vi "Get Startup Requirements.vi"(8 "error in (no error)":errorcluster, 10 "Startup Component":T1={"title"="", "description"="", "ID"="", "version"="", "component type"=4} {"component type" items=["standard", "hidden", "system", "unknown", "startup", "image", "essential"]}, 11 "Session in":refnum<k21>) -> (0 "error out":errorcluster, 1 "Software Set":T3 {"information"."component type" items=["standard", "hidden", "system", "unknown", "startup", "image", "essential"]; "items"."component type" items=["standard", "hidden", "system", "unknown", "startup", "image", "essential"]; "add-ons"."component type" items=["standard", "hidden", "system", "unknown", "startup", "image", "essential"]}, 2 "Dependencies":T4[](array[typedef]) {"dependee"."component type" items=["standard", "hidden", "system", "unknown", "startup", "image", "essential"]; "depender"."component type" items=["standard", "hidden", "system", "unknown", "startup", "image", "essential"]}, 3 "Session out":refnum<k21>)   [LabVIEW 2017, in "nisyscfg.lvlib"]
uses:
  <vilib>/nisyscfg/nisyscfg.lvlib
  <vilib>/nisyscfg/Broken Dependency 1.2.ctl
  <vilib>/nisyscfg/Software 1.2.ctl
  <vilib>/nisyscfg/Component Type.ctl
  <vilib>/nisyscfg/Software Set 1.2.ctl
  <vilib>/nisyscfg/Component Types.ctl
panel:
  out "Visibility Type":u32
  out "Type":u32
  out "Number of Items":i32
  out "Items":u64
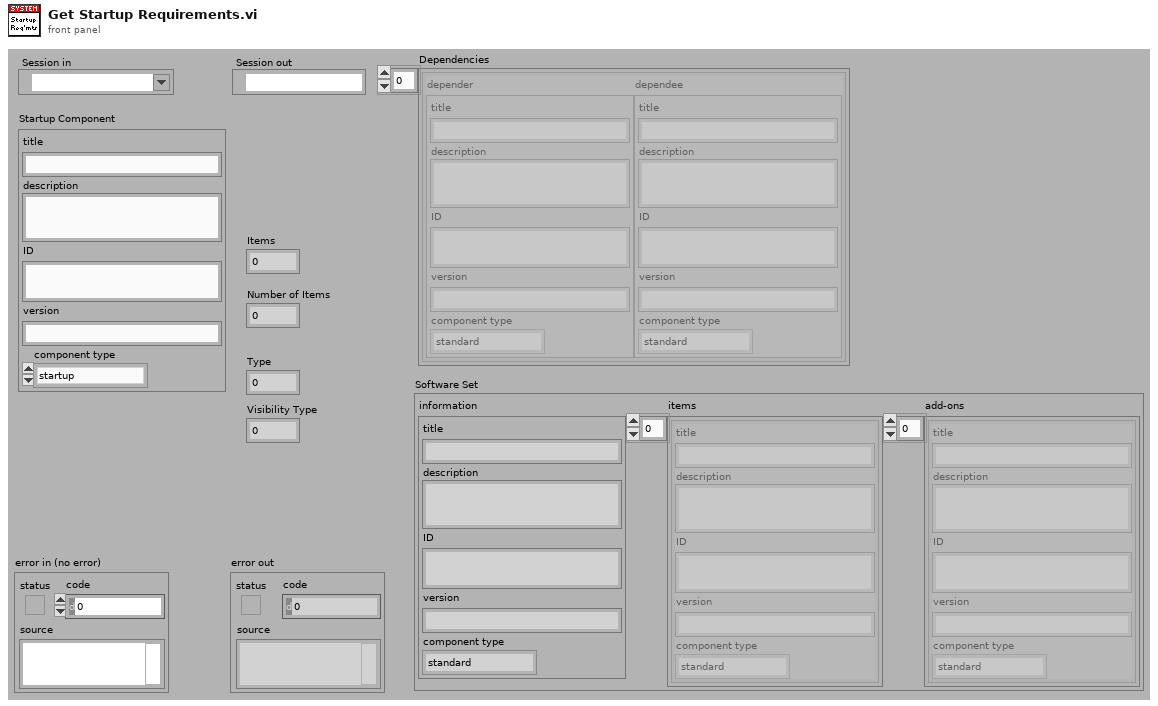
[diagram p1: front panel]
types:
  T1 = typedef "nisyscfg.lvlib/Software 1.2.ctl" = cluster{"title":string, "description":string, "ID":string, "version":string, "component type":T2}
  T2 = typedef "nisyscfg.lvlib/Component Type.ctl" = u32
  T3 = typedef "nisyscfg.lvlib/Software Set 1.2.ctl" = cluster{"information":T1, "items":T1[], "add-ons":T1[]}
  T4 = typedef "nisyscfg.lvlib/Broken Dependency 1.2.ctl" = cluster{"depender":T1, "dependee":T1}
  T5 = typedef "nisyscfg.lvlib/Component Types.ctl" = u32
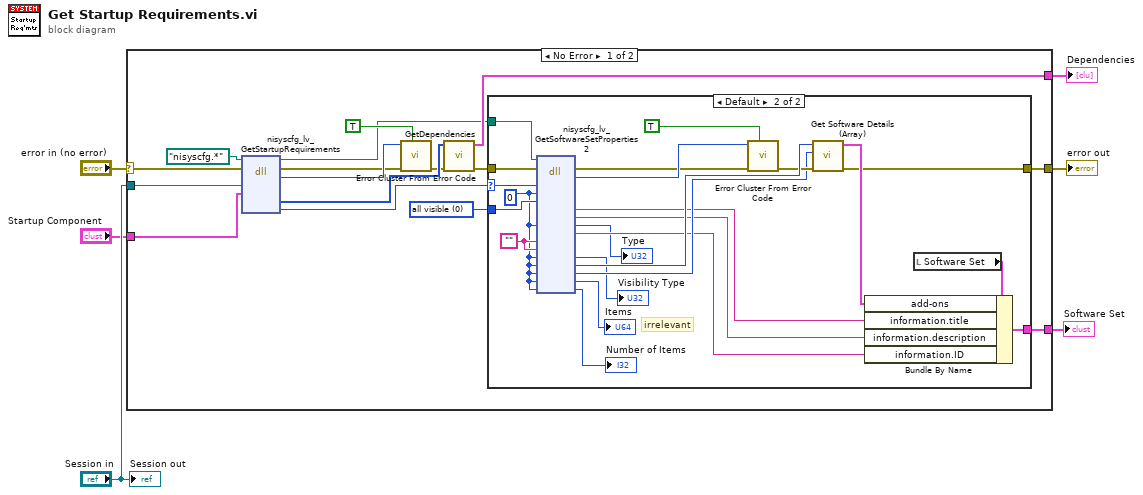
[diagram p0: block diagram]
diagram:
  n1 = case shown="No Error" "error in (no error)" {
    selector: "error in (no error)" -> [w20 w47]
    tunnel: [w11 w47] -> w4
    tunnel: "Session in" -> [w19 _]
    tunnel: [w14 _] -> w3
    tunnel: [w13 _] -> w2
    tunnel: "Startup Component" -> [w7 _]
    frame No Error {
      w8 = T5 0 items=["all visible", "all including hidden"] ("item types (visible only)")
      n2 = dll-call lib="nisyscfg.*" fn="nisyscfg_lv_GetStartupRequirements" label="GetStartupRequirements"(path in=path "nisyscfg.*", error in=w20, "system"=w19, "applicationInfo"=w7) -> (path out=w10:path, error out=w21:errorcluster, "result"=w22:i32, "components"=w16:u64[], "softwareSet"=w9:u64)  [unwired: 5 in]
      n3 = call <vilib>:"Error Cluster From Error Code.vi"("show call chain? (False)"=TRUE, "error in (no error)"=w21, "error code (0)"=w22) -> ("error out"=w15:errorcluster)  [unwired: 6 in]
      n4 = call <vilib>:"GetDependencies.vi"("error in (no error)"=w15, "Enumerator in"=w16) -> ("error out"=w12:errorcluster, "Dependencies"=w14:T4[])  [unwired: 8 in]
      n5 = case shown="Default" w9 {
        selector: w9 -> [_ w37]
        tunnel: w12 -> [w23 w46]
        tunnel: [w23 w27] -> w11
        tunnel: [_ w43] -> w13
        tunnel: w10 -> [_ w42]
        tunnel: w8 -> [_ w32]
        frame 0 {
        }
        frame Default {
          w26 = ""
          w25 = u8 0 ("includeAddOnDeps")
          # "irrelevant"
          n6 = dll-call lib="nisyscfg.*" fn="nisyscfg_lv_GetSoftwareSetProperties2" label="GetSoftwareSetProperties2"(path in=w42, error in=w46, "set"=w37, "includeAddOnDeps"=w25, "includeTypes"=w32, "type"=w25, "groupID"=w26, "version"=w26, "visibleType"=w25, "addons"=w25, "numAddons"=w25, "items"=w25, "numItems"=w25) -> (error out=w44:errorcluster, "result"=w45:i32, "title"=w34:string, "description"=w35:string, "type"=→"Type":u32, "ID"=w33:string, "visibleType"=→"Visibility Type":i32, "addons"=w40:u64, "numAddons"=w36:i32, "items"=→"Items":u64, "numItems"=→"Number of Items":i32)  [unwired: 9 in, 1 out]
          n7 = call <vilib>:"Error Cluster From Error Code.vi"("show call chain? (False)"=TRUE, "error in (no error)"=w44, "error code (0)"=w45) -> ("error out"=w39:errorcluster)  [unwired: 6 in]
          n8 = call <vilib>:"Get Software Details (Array).vi"("error in (no error)"=w39, "Number of Elements"=w36, "Enumerator in"=w40) -> ("error out"=w27:errorcluster, "Software Components"=w31:T1[])  [unwired: 7 in]
          n9 = local read "Software Set"() -> (w38:T3)
          n10 = Bundle By Name(cluster=w38, "add-ons"=w31, "information.title"=w34, "information.description"=w35, "information.ID"=w33) -> (w43:T3)
        }
      }
    }
    frame Error {
    }
  }
  "error out" <- w4
  "Dependencies" <- w3
  "Software Set" <- w2
  "Session out" <- "Session in"
